vi "03_Buttons.vi"() -> ()   [LabVIEW 2020]
panel:
  in  "Padding (px)":i32=5
  in  "Horizontal?":bool
  in  "Visible?":bool[](array[boolean])=[TRUE, TRUE, TRUE, TRUE]
  in  "Arrow Right":bool
  in  "Arrow Left":bool
  in  "Rotate Right":bool
  in  "Rotate Left":bool
  # "Configuration"
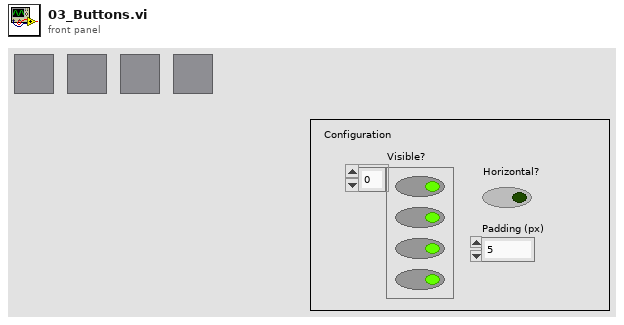
[diagram p1: front panel]
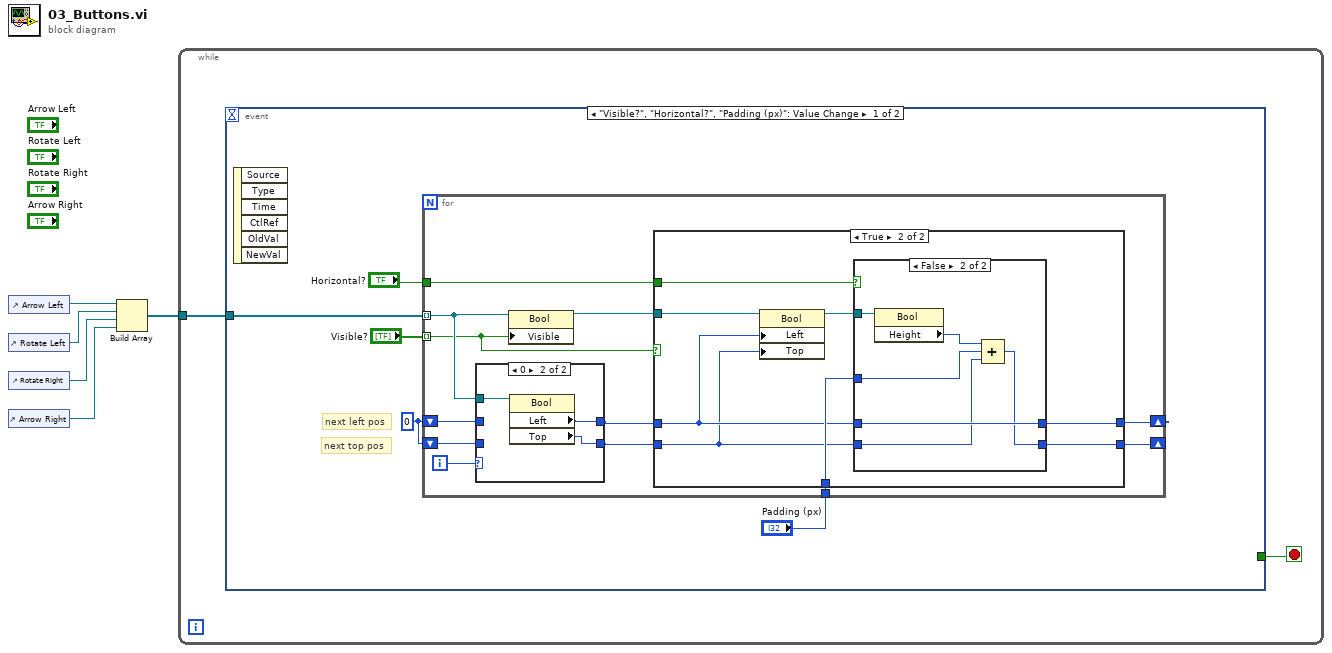
[diagram p0: block diagram]
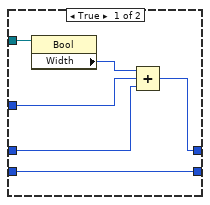
[diagram p3: hidden frame]
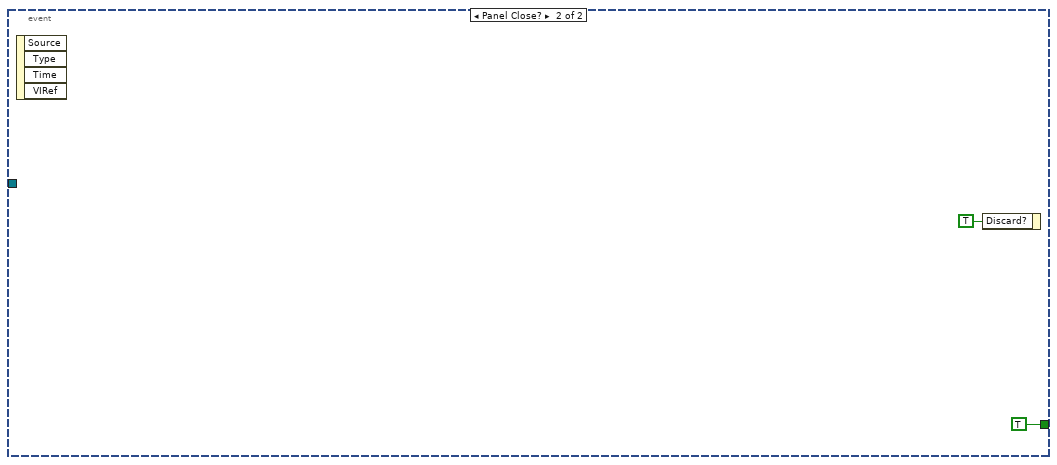
[diagram p5: hidden frame]
diagram:
  n1 = control-ref of="Arrow Left"() -> (w5:refnum<vi>)
  n2 = control-ref of="Rotate Left"() -> (w4:refnum<vi>)
  n3 = control-ref of="Rotate Right"() -> (w3:refnum<vi>)
  n4 = control-ref of="Arrow Right"() -> (w2:refnum<vi>)
  n5 = Build Array(w5, w4, w3, w2) -> (w1:refnum<vi>[])
  n6 = while {
    tunnel: w1 -> [w7]
    stop <- w6 stop-if-true
    n7 = event shown="[0] \"Visible?\", \"Horizontal?\", \"Padding (px)\": Value Change" {
      selector: _ -> [_ _]
      dyn-events: _ -> [_ _]
      timeout: _ -> [_ _]
      tunnel: w7 -> [w12 _]
      tunnel: [_ TRUE] -> w6
      event "Visible?", "Horizontal?", "Padding (px)": Value Change {
        w11 = 0 ("Left")
        # "next top pos"
        # "next left pos"
        n8 = event-data() -> ()  [unwired: 1 in, 6 out]
        n9 = for {
          tunnel: w12 -> [w21] mode=indexing
          shift-right: [w16] -> _
          shift-left: w11 -> [w23]
          shift-right: [w15] -> _
          shift-left: w11 -> [w22]
          tunnel: "Visible?" -> [w20] mode=indexing
          tunnel: "Horizontal?" -> [w14]
          tunnel: "Padding (px)" -> [w13]
          i -> [w24]
          n10 = case shown="0" w24 {
            tunnel: w21 -> [_ w51]
            tunnel: [w48 w50] -> w18
            tunnel: [w47 w49] -> w17
            tunnel: w23 -> [w48 _]
            tunnel: w22 -> [w47 _]
            frame Default {
            }
            frame 0 {
              n11 = property class="Bool"(reference=w51) -> ("Left"=w50:i32, "Top"=w49:i32)  [unwired: 1 in, 2 out]
            }
          }
          n12 = property class="Bool"(reference=w21, "Visible"=w20) -> (reference out=w19:refnum<vi>)  [unwired: 1 in, 1 out]
          n13 = case shown="True" w20 {
            tunnel: w19 -> [_ w34]
            tunnel: w18 -> [w26 w29]
            tunnel: w17 -> [w25 w27]
            tunnel: [w26 w30] -> w16
            tunnel: [w25 w28] -> w15
            tunnel: w14 -> [_ w33]
            tunnel: w13 -> [_ w31]
            frame False {
            }
            frame True {
              n14 = property class="Bool"(reference=w34, "Left"=w29, "Top"=w27) -> (reference out=w32:refnum<vi>)  [unwired: 1 in, 1 out]
              n15 = case shown="False" w33 {
                tunnel: w32 -> [w40 w46]
                tunnel: w31 -> [w37 w44]
                tunnel: [w35 w43] -> w30
                tunnel: w29 -> [w36 w43]
                tunnel: [w38 w42] -> w28
                tunnel: w27 -> [w38 w41]
                frame True {
                  n16 = property class="Bool"(reference=w40) -> ("Width"=w39:u32)  [unwired: 1 in, 2 out]
                  n17 = Compound Arithmetic op=ADD(w39, w37, w36) -> (w35:u32)
                }
                frame False {
                  n18 = property class="Bool"(reference=w46) -> ("Height"=w45:u32)  [unwired: 1 in, 2 out]
                  n19 = Compound Arithmetic op=ADD(w45, w44, w41) -> (w42:u32)
                }
              }
            }
          }
        }
      }
      event Panel Close? {
        n20 = event-data() -> ()  [unwired: 1 in, 4 out]
        n21 = event-data("Discard?"=TRUE) -> ()  [unwired: 1 in, 1 out]
      }
    }
  }
